vi "YtScuffCountTest.vi"(11 "YTESTER测试数据":T1 caption="不要修改！") -> (3 "YTESTER结论":T2)   [LabVIEW 2017]
doc: "VIDescription=超过一定测试次数后，需要更换配件。通过此步骤管控。"
uses:
  YtCommon.lvlibp/yt`Step StepBaseInput.ctl
  YtCommon.lvlibp/yt`Step StepResult.ctl
  YtCommon.lvlibp/yt`Step TestData.ctl
  YtCommon.lvlibp/yt`Step System Queue.ctl
  Step`s VIs/YYLLGeneric/variable_W.ctl
  YtCommon.lvlibp/yt`Data-Ytester Type Data.ctl
  c8cbc2a2-276b-4a9c-a0cd-9eed75608cff.vi
  <vilib>/Utility/error.llb/Clear Errors.vi
  YtCommon.lvlibp/yt`varSystemlib IO Read Variable.vi
  YtCommon.lvlibp
panel:
  in  "YTESTER开放参数":cluster{"YTESTER_BaseInput":T3, "最大次数":i32}={"YTESTER_BaseInput"={"isTest"=TRUE, "isSkip"=FALSE, "StepName"="损耗计数", "OnPass"=enum."Next", "OnFail"=enum."Terminate", "ReTestNumber"=0.0}, "最大次数"=1000}
  # "损耗计数"
  # "作为一个Test，显示本次次数和最大次数\n当测试超过最大次数默认终止测试输出Fail!\n\n如何复位？修改为0或删除YtScuffCount变量！"
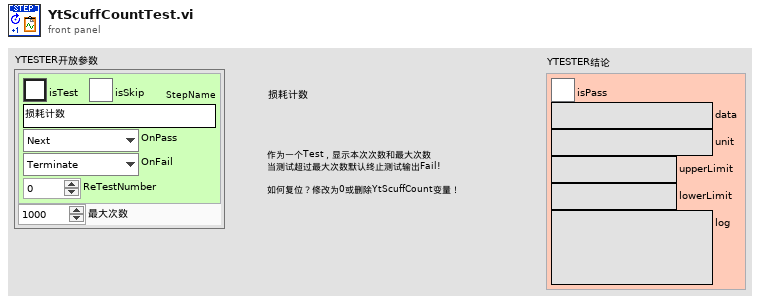
[diagram p1: front panel]
types:
  T1 = typedef "YtCommon.lvlibp/yt`Step TestData.ctl" = cluster{"Socket(From1)":i32, "SN":refnum<notifier>, "StopFlagRef":refnum<notifier>, "YT System Queue":refnum<queue>}
  T2 = typedef "YtCommon.lvlibp/yt`Step StepResult.ctl" = cluster{"isPass":bool, "data":string, "unit":string, "upperLimit":string, "lowerLimit":string, "log":string}
  T3 = typedef "YtCommon.lvlibp/yt`Step StepBaseInput.ctl" = cluster{"isTest":bool, "isSkip":bool, "StepName":string, "OnPass":enum16{"Next", "ToOVER", "Terminate"}, "OnFail":enum16{"Next", "ToOVER", "Terminate"}, "ReTestNumber":dbl}
  T4 = typedef "variable_W.ctl" = cluster{"YT_TYPE":T5, "TypeData":string[], "Tips":string}
  T5 = typedef "YtCommon.lvlibp/yt`Data-Ytester Type Data.ctl" = enum16{"NULL", "NUM", "BOOL", "TXT", "ENUM", "TIME", "PATH", "VISA", "COMBO", "ColorBox", "RadioBtn", "Array_NUM", "Array_BOOL", "Array_TXT", "Array_ENUM", "Array_PATH", "Array_COMBO"}
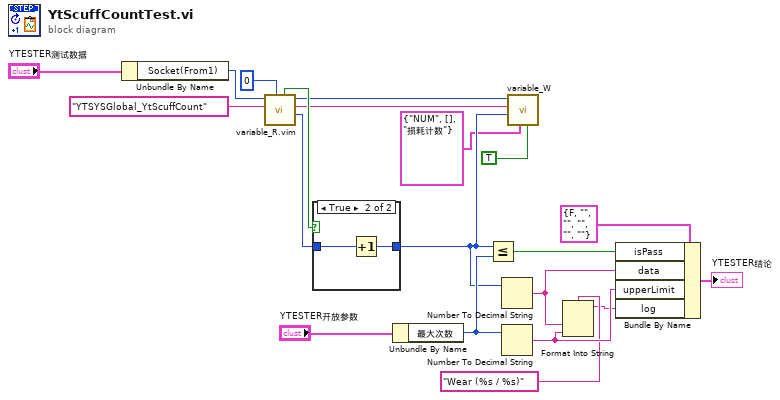
[diagram p0: block diagram]
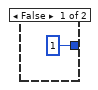
[diagram p2: hidden frame]
diagram:
  n1 = Unbundle By Name("YTESTER测试数据") -> ("Socket(From1)"=w8:i32)
  n2 = call "variable_R.vim"("type"=0, "待获取变量名称"="YTSYSGlobal_YtScuffCount" ("format string"), "函数池名称"=w8) -> ("value"=w13:i32, "待获取变量名out"=w11:string, "函数池名称out"=w12:i32, "found?"=w14:bool)  [unwired: 4 in, 1 out]
  n3 = case shown="True" w14 {
    tunnel: [1 w22] -> w7
    tunnel: w13 -> [_ w23]
    frame False {
    }
    frame True {
      n4 = Increment(x=w23) -> (x+1=w22:i32)
    }
  }
  n5 = Unbundle By Name("YTESTER开放参数") -> ("最大次数"=w9:i32)
  n6 = Less Or Equal?(x=w7, y=w9) -> (x <= y?=w10:bool)
  n7 = Number To Decimal String(number=w7) -> (decimal integer string=w4:string)  [unwired: 1 in]
  n8 = Number To Decimal String(number=w9) -> (decimal integer string=w3:string)  [unwired: 1 in]
  n9 = call "variable_W.vi"("永久生成在本地（F）"=TRUE, "附加的Information"=T4 {"YT_TYPE"=enum."NUM", "TypeData"=[], "Tips"="损耗计数"}, "待写入池的输入控件"=w7, "待写入池变量名称"=w11, "函数池名称 in"=w12) -> ()  [unwired: 4 in, 3 out]
  n10 = Format Into String(format string="Wear (%s / %s)", w4, w3) -> (resulting string=w1:string)  [unwired: 2 in, 1 out]
  n11 = Bundle By Name(cluster=T2 {"isPass"=FALSE, "data"="", "unit"="", "upperLimit"="", "lowerLimit"="", "log"=""} ("Result"), "isPass"=w10, "data"=w4, "upperLimit"=w3, "log"=w1) -> (→"YTESTER结论":T2)
